vi "Fixated Autoadjust.vi"(10 "Input":variant, 11 "Data":T1) -> (2 "Fixated":bool, 3 "Adjustment":dbl[](array[numeric]))   [LabVIEW 2011]
uses:
  Z:/libraries/Labview/Core SubVIs/Controls/TYPE - Analog Data.ctl
  Z:/libraries/Labview/Trial Based Experiment/TYPE - State triggers.ctl
  <vilib>/imath/engines/lvmath2/RunTimeEngine/ErrorHandling/NIMS_Finalize Error.vi
  <vilib>/imath/engines/lvmath2/RunTimeEngine/NodeEndStatement/NIMS_NodeEndStatement_Output.vi
  <instcachedir>/0/NIMS_NodeEndStatement_Output_53EC0D466D134D7ABD903AC30B43404B.lvgen/NIMS_NodeEndStatement_Output_53EC0D466D134D7ABD903AC30B43404B_009.vi
  <vilib>/imath/engines/lvmath2/RunTimeEngine/BuiltInFunctions/sum/NIMS_sum(GV).vi
  <instcachedir>/0/NIMS_sum(GV)_67F5EC36BC034E54A6BEC5B0673C00E5.lvgen/NIMS_sum(GV)_67F5EC36BC034E54A6BEC5B0673C00E5_000.vi
  <vilib>/imath/engines/lvmath2/RunTimeEngine/ArithmeticOperatorToken/NIMS_ArithmeticOperator_multmx(RV,CV)-internal.vi
  <instcachedir>/0/NIMS_ArithmeticOperator_multmx(RV,CV)-internal_26C0DCAD7F024225968CB0639EC17D76.lvgen/NIMS_ArithmeticOperator_multmx(RV,CV)-internal_26C0DCAD7F024225968CB0639EC17D76_006.vi
  <vilib>/imath/engines/lvmath2/RunTimeEngine/BuiltInFunctions/abs/NIMS_abs(signed).vi
  <instcachedir>/0/NIMS_abs(signed)_C4FCB8E6058B49B797C7C8D53CA5F6EC.lvgen/NIMS_abs(signed)_C4FCB8E6058B49B797C7C8D53CA5F6EC_002.vi
  <vilib>/imathl/engines/lvmath/Functions/Error Handling/Create Error.vi
  <vilib>/Analysis/baseanly.llb/Unimode.vi
  <vilib>/Analysis/NI_AALBase.lvlib
  Z:/libraries/Labview/Core SubVIs/Core SubVIs.lvlib
panel:
  in  "incTargRad":dbl=100.0
  out "Max. running window size":i32=1000
  in  "Learning rate":dbl=0.0003
  in  "Minimum for update":i32=40
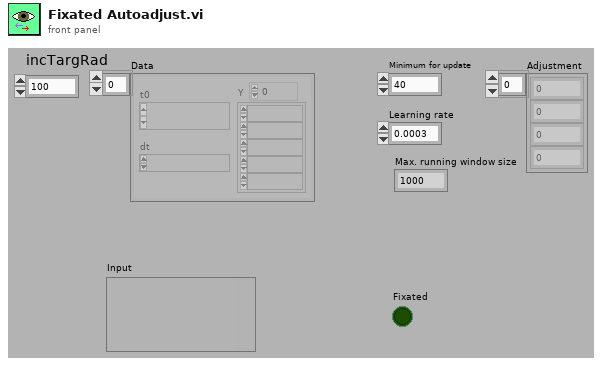
[diagram p1: front panel]
types:
  T1 = typedef "Core SubVIs.lvlib/TYPE - Analog Data.ctl" = waveform(dbl)[]
  T2 = typedef "TYPE - State triggers.ctl" = enum16{"Start Session", "Start Trial", "Intertrial", "Acquire Fixation", "Delay Period", "Response Period", "Reward", "Abort Trial", "End Trial"}
  T3 = cluster{"Trial Type":i32, "Joystick Threshold":dbl, "Fixation Radius":dbl, "Left Target":dbl[][], "Right Target":dbl[][], "Target Radius":dbl, "Trigger":T2}
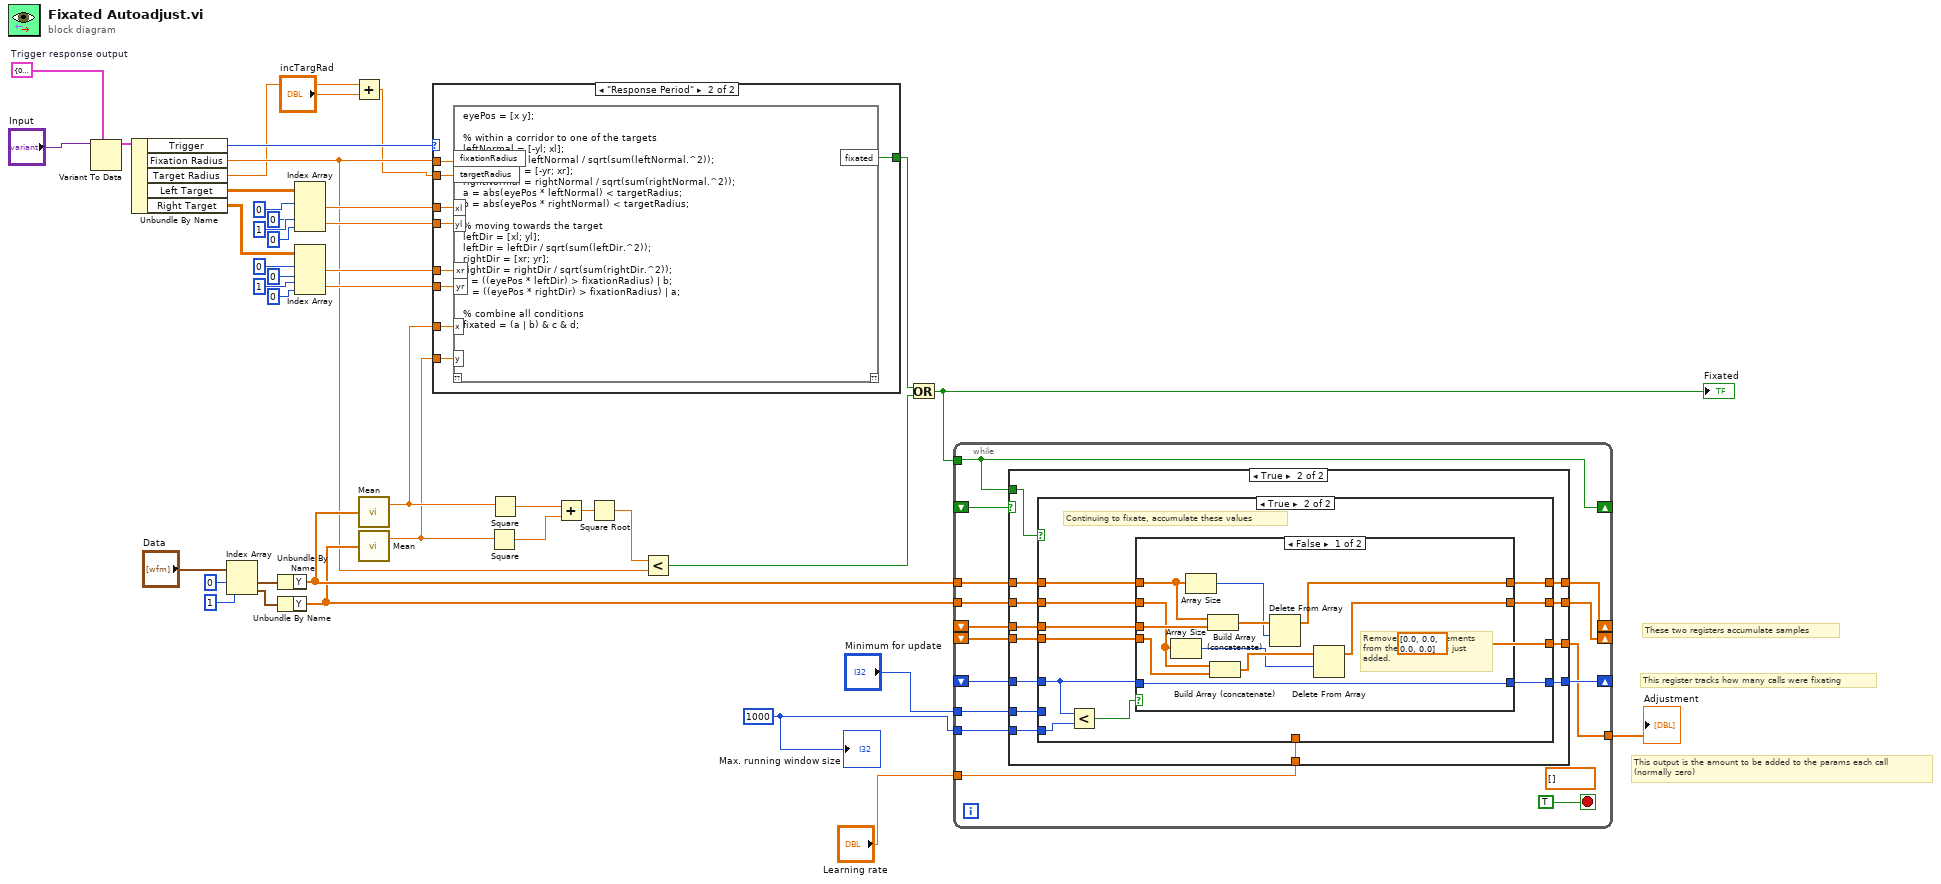
[diagram p0: block diagram]
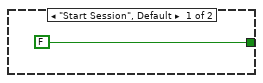
[diagram p2: hidden frame]
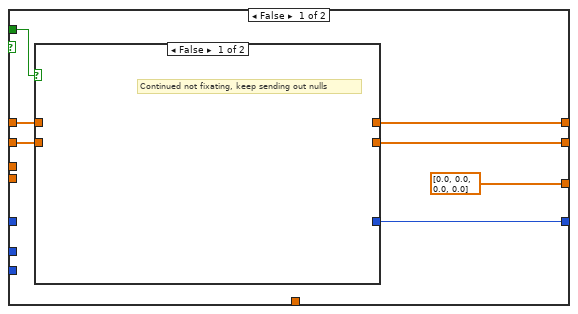
[diagram p3: hidden frame]
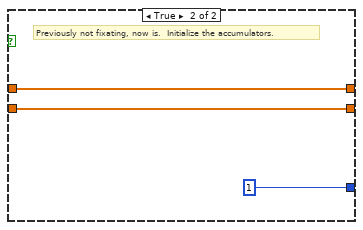
[diagram p4: hidden frame]
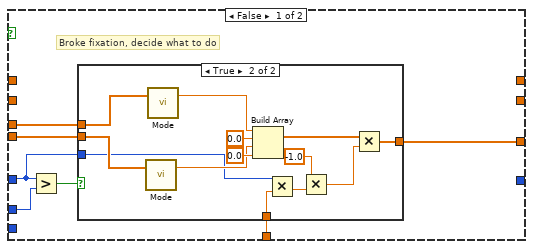
[diagram p5: hidden frame]
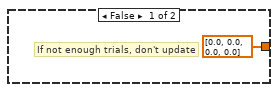
[diagram p6: hidden frame]
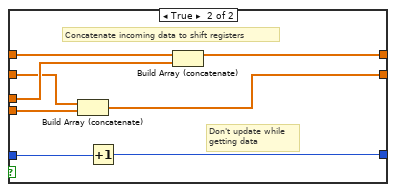
[diagram p7: hidden frame]
diagram:
  w31 = T3 {"Trial Type"=0, "Joystick Threshold"=0.0, "Fixation Radius"=0.0, "Left Target"=[], "Right Target"=[], "Target Radius"=0.0, "Trigger"=enum."End Trial"}  # Trigger response output
  w34 = 1000
  # "This output is the amount to be added to the params each call\n(normally zero)"
  # "These two registers accumulate samples"
  # "This register tracks how many calls were fixating"
  n1 = Variant To Data(type=w31, Variant="Input") -> (data=w32:T3)  [unwired: 1 in, 1 out]
  n2 = Unbundle By Name(w32) -> ("Trigger"=w30:T2, "Fixation Radius"=w7:dbl, "Target Radius"=w3:dbl, "Left Target"=w21:dbl[][], "Right Target"=w20:dbl[][])
  n3 = Index Array(array="Data", index #1=0 ("index"), index #2=1 ("index")) -> (element #1=w39:waveform(dbl), element #2=w38:waveform(dbl))
  n4 = Unbundle By Name(w39) -> ("Y"=w15:dbl[])
  n5 = Unbundle By Name(w38) -> ("Y"=w14:dbl[])
  n6 = Index Array(array=w21, index (row) #1=0 ("index"), index (col) #1=0 ("disabled index (col)"), index (row) #2=1 ("index"), index (col) #2=0 ("disabled index (col)")) -> (element #1=w19:dbl, element #2=w18:dbl)
  n7 = Index Array(array=w20, index (row) #1=0 ("index"), index (col) #1=0 ("disabled index (col)"), index (row) #2=1 ("index"), index (col) #2=0 ("disabled index (col)")) -> (element #1=w17:dbl, element #2=w16:dbl)
  n8 = Add(x=w3, y="incTargRad") -> (x+y=w2:dbl)
  n9 = call <vilib>:"Mean.vi"("X"=w15) -> ("mean"=w9:dbl)  [unwired: 1 out]
  n10 = call <vilib>:"Mean.vi"("X"=w14) -> ("mean"=w8:dbl)  [unwired: 1 out]
  n11 = case shown="\"Response Period\"" w30 {
    tunnel: w7 -> [_ w51]
    tunnel: [FALSE w46] -> w6
    tunnel: w2 -> [_ w52]
    tunnel: w19 -> [_ w50]
    tunnel: w18 -> [_ w49]
    tunnel: w17 -> [_ w48]
    tunnel: w16 -> [_ w47]
    tunnel: w9 -> [_ w45]
    tunnel: w8 -> [_ w44]
    frame "Start Session", Default {
    }
    frame "Response Period" {
      n12 = mathscript code="eyePos = [x y];\n\n% within a corridor to one of the targets\nleftNormal = [-yl; xl];\nleftNormal = leftNormal / sqrt(sum(leftNormal.^2));\nrightNormal = [-yr; xr];\nrightNormal = rightNormal / sqrt(sum(rightNormal.^2));\na = abs(eyePos * leftNormal) < targetRadius;\nb = abs(eyePos * rightNormal) < targetRadius;\n\n% moving towards the target\nleftDir = [xl; yl];\nleftDir = leftDir / sqrt(sum(leftDir.^2));\nrightDir = [xr; yr];\nrightDir = rightDir / sqrt(sum(rightDir.^2));\nc = ((eyePos * leftDir) > fixationRadius) | b;\nd = ((eyePos * rightDir) > fixationRadius) | a;\n\n% combine all conditions\nfixated = (a | b) & c & d;"("xl"=w50, "yl"=w49, "xr"=w48, "yr"=w47, "fixationRadius"=w51, "targetRadius"=w52, "x"=w45, "y"=w44) -> ("fixated"=w46:bool)  [unwired: 1 in, 1 out]
    }
  }
  n13 = Square(x=w8) -> (x^2=w10:dbl)
  n14 = Square(x=w9) -> (x^2=w11:dbl)
  n15 = Add(x=w11, y=w10) -> (x+y=w13:dbl)
  n16 = Square Root(x=w13) -> (sqrt(x)=w12:dbl)
  n17 = Less?(x=w12, y=w7) -> (x < y?=w5:bool)
  n18 = Or(x=w6, y=w5) -> (x .or. y?=w4:bool)
  "Fixated" <- w4
  n19 = while {
    tunnel: w4 -> [w235]
    shift-right: [w235] -> _
    shift-left: _ -> [w248]
    shift-right: [w247] -> _
    shift-left: _ -> [w242]
    tunnel: w14 -> [w246]
    tunnel: w15 -> [w245]
    shift-right: [w237] -> _
    shift-left: _ -> [w244]
    shift-right: [w236] -> _
    shift-left: _ -> [w243]
    tunnel: "Minimum for update" -> [w241]
    tunnel: "Learning rate" -> [w240]
    tunnel: [w239] -> w35
    tunnel: w34 -> [w238]
    stop <- TRUE stop-if-true
    (unwired) dbl[] []
    n20 = case shown="True" w248 {
      tunnel: w235 -> [w256 w264]
      tunnel: [w255 w265] -> w247
      tunnel: w246 -> [w254 w268]
      tunnel: w245 -> [w253 w272]
      tunnel: [w252 w270] -> w237
      tunnel: [w251 w267] -> w236
      tunnel: w244 -> [_ w271]
      tunnel: w243 -> [_ w269]
      tunnel: w242 -> [_ w266]
      tunnel: w241 -> [_ w263]
      tunnel: w240 -> [_ w262]
      tunnel: [dbl[] [0.0, 0.0, 0.0, 0.0] w261] -> w239
      tunnel: w238 -> [_ w260]
      frame False {
        n21 = case shown="False" w256 {
          tunnel: [_ 1] -> w255
          tunnel: w254 -> [_ w257]
          tunnel: w253 -> [_ w258]
          tunnel: [_ w258] -> w252
          tunnel: [_ w257] -> w251
          frame False {
            # "Continued not fixating, keep sending out nulls"
          }
          frame True {
            # "Previously not fixating, now is.  Initialize the accumulators."
          }
        }
      }
      frame True {
        n22 = case shown="True" w264 {
          tunnel: w272 -> [_ w304]
          tunnel: w271 -> [w277 w303]
          tunnel: [_ w296] -> w270
          tunnel: w269 -> [w276 w302]
          tunnel: w268 -> [_ w301]
          tunnel: [_ w295] -> w267
          tunnel: w266 -> [w274 w294]
          tunnel: [_ w300] -> w265
          tunnel: w263 -> [w279 _]
          tunnel: w262 -> [w275 _]
          tunnel: [w273 dbl[] [0.0, 0.0, 0.0, 0.0]] -> w261
          tunnel: w260 -> [_ w298]
          frame False {
            # "Broke fixation, decide what to do"
            n23 = Greater?(x=w274, y=w279) -> (0:w278:bool)
            n24 = case shown="True" w278 {
              tunnel: w277 -> [_ w293]
              tunnel: w276 -> [_ w292]
              tunnel: w275 -> [_ w286]
              tunnel: w274 -> [_ w285]
              tunnel: [dbl[] [0.0, 0.0, 0.0, 0.0] w281] -> w273
              frame False {
                # "If not enough trials, don't update"
              }
              frame True {
                n25 = call-poly <vilib>:"Mode.vi"("X"=w292) -> ("mode"=w288:dbl)  [unwired: 1 in, 1 out]
                n26 = call-poly <vilib>:"Mode.vi"("X"=w293) -> ("mode"=w291:dbl)  [unwired: 1 in, 1 out]
                n27 = Build Array(w291, 0.0 ("element"), w288, 0.0 ("element")) -> (w287:dbl[])
                n28 = Multiply(x=w285, y=w286) -> (x*y=w284:dbl)
                n29 = Multiply(x=-1.0, y=w284) -> (x*y=w282:dbl)
                n30 = Multiply(x=w287, y=w282) -> (x*y=w281:dbl[])
              }
            }
          }
          frame True {
            # "Continuing to fixate, accumulate these values"
            n31 = Less?(x=w294, y=w298) -> (x < y?=w297:bool)
            n32 = case shown="False" w297 {
              tunnel: w304 -> [w313 w323]
              tunnel: w303 -> [w314 w322]
              tunnel: [w310 w321] -> w296
              tunnel: w302 -> [w309 w320]
              tunnel: w301 -> [w308 w319]
              tunnel: [w305 w318] -> w295
              tunnel: [w315 w317] -> w300
              tunnel: w294 -> [w315 w316]
              frame False {
                # "Remove as many elements\nfrom the array as we just\nadded."
                n33 = Array Size(array=w308) -> (size(s)=w306:i32)
                n34 = Array Size(array=w313) -> (size(s)=w311:i32)
                n35 = Build Array (concatenate)(w313, w314) -> (w312:dbl[])
                n36 = Build Array (concatenate)(w308, w309) -> (w307:dbl[])
                n37 = Delete From Array(array=w312, length=w311) -> (array with subset deleted=w310:dbl[])  [unwired: 1 in, 1 out]
                n38 = Delete From Array(array=w307, length=w306) -> (array with subset deleted=w305:dbl[])  [unwired: 1 in, 1 out]
              }
              frame True {
                # "Concatenate incoming data to shift registers"
                # "Don't update while\ngetting data"
                n39 = Build Array (concatenate)(w319, w320) -> (w318:dbl[])
                n40 = Increment(x=w316) -> (x+1=w317:i32)
                n41 = Build Array (concatenate)(w323, w322) -> (w321:dbl[])
              }
            }
          }
        }
      }
    }
  }
  "Adjustment" <- w35
  "Max. running window size" <- w34
